vi "ErrorPfad.vi"(5 "Message In":string, 7 "Numeric":i32, 11 "error in (no error)":errorcluster) -> (6 "Message Out":string, 15 "error out":errorcluster)   [LabVIEW 2014, in "FH 55.lvlib"]
doc: "This VI checks the answer of the instrument of ERRORs. If they found the word ERROR in the answer the VI gives ERROR back."
uses:
  FH 55.lvlib
panel:
  in  "error in (no error) 2":errorcluster
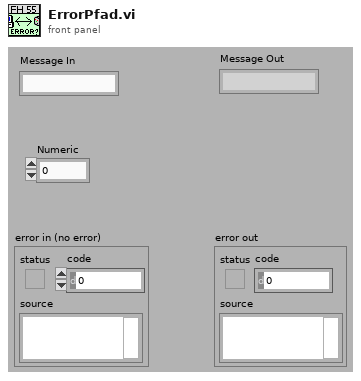
[diagram p1: front panel]
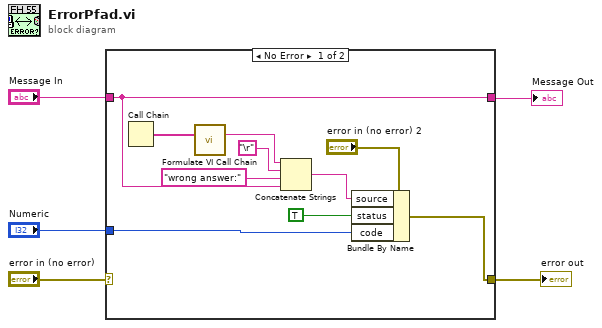
[diagram p0: block diagram]
diagram:
  n1 = case shown="No Error" "error in (no error)" {
    selector: "error in (no error)" -> [_ w16]
    tunnel: [w8 w16] -> w4
    tunnel: "Message In" -> [w7 w17]
    tunnel: [w7 w17] -> w2
    tunnel: "Numeric" -> [w6 _]
    frame No Error {
      n2 = Call Chain() -> (call chain=w12:string[])
      n3 = call "Formulate VI Call Chain.vi"("Call Chain"=w12) -> ("String Out"=w11:string)  [unwired: 14 in]
      n4 = Concatenate Strings(w11, "\r", "wrong answer:", w7) -> (w13:string)
      n5 = Bundle By Name(cluster="error in (no error) 2", "source"=w13, "status"=TRUE, "code"=w6) -> (w8:errorcluster)
    }
    frame Error {
    }
  }
  "Message Out" <- w2
  "error out" <- w4
